vi "FTW-WebService-Respond.vi"(0 "FTW Web Request":refnum<class "FTW-WebService.lvclass">, 5 "HTTP Response Code":T1=200 items=["100 Continue"=100, "101 Switching Protocols"=101, "200 OK"=200, "201 Created"=201, "202 Accepted"=202, "203 Non-Authoritative Information"=203, "204 No Content"=204, "205 Reset Content"=205, "206 Partial Content"=206, "300 Multiple Choices"=300, "301 Moved Permanently"=301, "302 Found"=302, "303 See Other"=303, "304 Not Modified"=304, "305 Use Proxy"=305, "306 (Unused)"=306, "307 Temporary Redirect"=307, "400 Bad Request"=400, "401 Unauthorized"=401, "402 Payment Required"=402, "403 Forbidden"=403, "404 Not Found"=404, "405 Method Not Allowed"=405, "406 Not Acceptable"=406, "407 Proxy Authentication Required"=407, "408 Request Timeout"=408, "409 Conflict"=409, "410 Gone"=410, "411 Length Required"=411, "412 Precondition Failed"=412, "413 Request Entity Too Large"=413, "414 Request-URI Too Long"=414, "415 Unsupported Media Type"=415, "416 Requested Range Not Satisfiable"=416, "417 Expectation Failed"=417, "500 Internal Server Error"=500, "501 Not Implemented"=501, "502 Bad Gateway"=502, "503 Service Unavailable"=503, "504 Gateway Timeout"=504, "505 HTTP Version Not Supported"=505], 7 "Response Body":string, 11 "error in":errorcluster) -> (4 "FTW Web Request out":refnum<class "FTW-WebService.lvclass">, 15 "error out":errorcluster)   [LabVIEW 2013, in "FTW-WebService.lvclass"]
uses:
  FTW-WebService.lvclass
  FTW-HTTP-ResponseCode.ctl
  FTW-WebService.lvclass/FTW-WebService.ctl
  FTW-WebService-Response.ctl
panel:
  # "Inputs"
  # "Outputs"
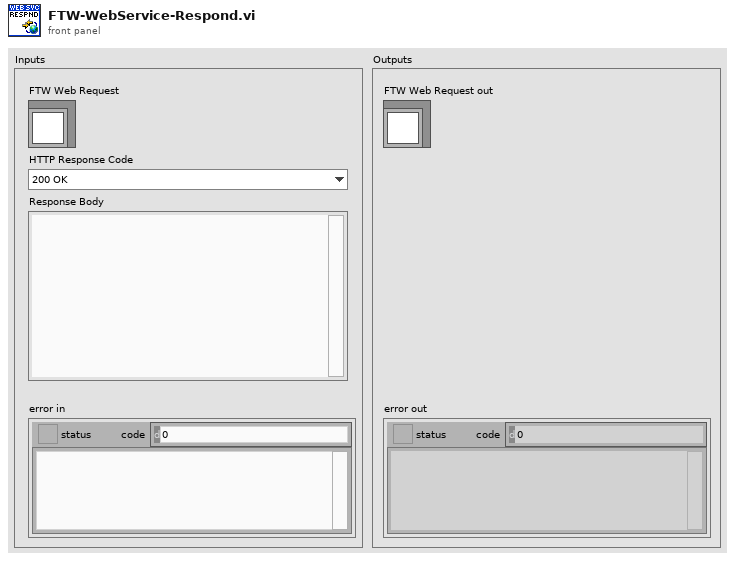
[diagram p1: front panel]
types:
  T1 = typedef "FTW-HTTP-ResponseCode.ctl" = i32
  T2 = typedef "FTW-WebService.lvclass/FTW-WebService-Response.ctl" = cluster{"HTTP Response Code":T1, "Response Body":string}
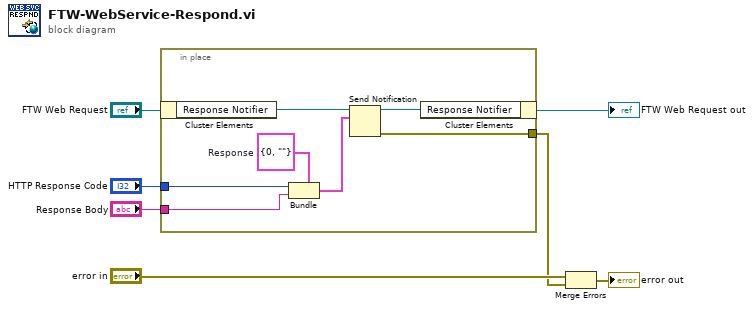
[diagram p0: block diagram]
diagram:
  n1 = in-place {
    in-place-border: "Response Body" -> [w12]
    in-place-border: "HTTP Response Code" -> [w13]
    in-place-border: [w11] -> w2
    w10 = T2 {"HTTP Response Code"=0, "Response Body"=""}  # Response
    n2 = in-place-cluster #1("FTW Web Request") -> ("Response Notifier"=w9:refnum<notifier>)
    n3 = Bundle(cluster=w10, "HTTP Response Code"=w13, "Response Body"=w12) -> (w8:T2)
    n4 = Send Notification(notification=w8, notifier=w9) -> (notifier out=w14:refnum<notifier>, error out=w11:errorcluster)  [unwired: 1 in]
    n5 = in-place-cluster #1("Response Notifier"=w14) -> (→"FTW Web Request out":refnum<class "FTW-WebService.lvclass">)
  }
  n6 = Merge Errors("error in", w2) -> (→"error out":errorcluster)
